vi "Find all vis in memory without documentation.vi"() -> ()   [LabVIEW 2010]
doc: "This .vi searches all .vi's in memory and returns the ones that do not have documentation. The .vis that are controls, in the .vi lib are ignored. The control on the front panel allows these .vis to be openned."
panel:
  in  "State":T1(ring)=enum."Minimized"
  out "Vis checked":i32(slide) scale=0.0..974.0
  in  "Open FPs of VI's without Documentation?":bool
  out "Total # without doc":i32
  out "Files without Documentation":string[](array[string])
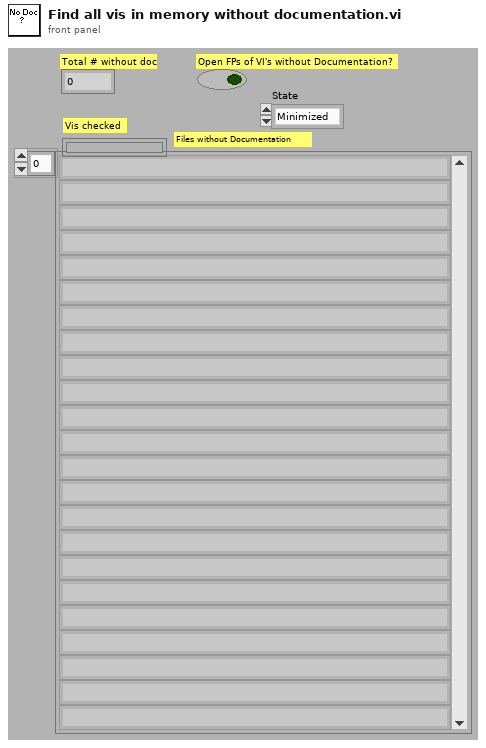
[diagram p1: front panel]
types:
  T1 = enum32{"Invalid", "Standard", "Closed", "Hidden", "Minimized", "Maximized"}
  T2 = enum32{"invalid VI type", "Standard VI", "Control VI", "Global VI", "Polymorphic VI", "Configuration VI", "SubSystem", "Facade VI", "Method VI", "Statechart Diagram VI"}
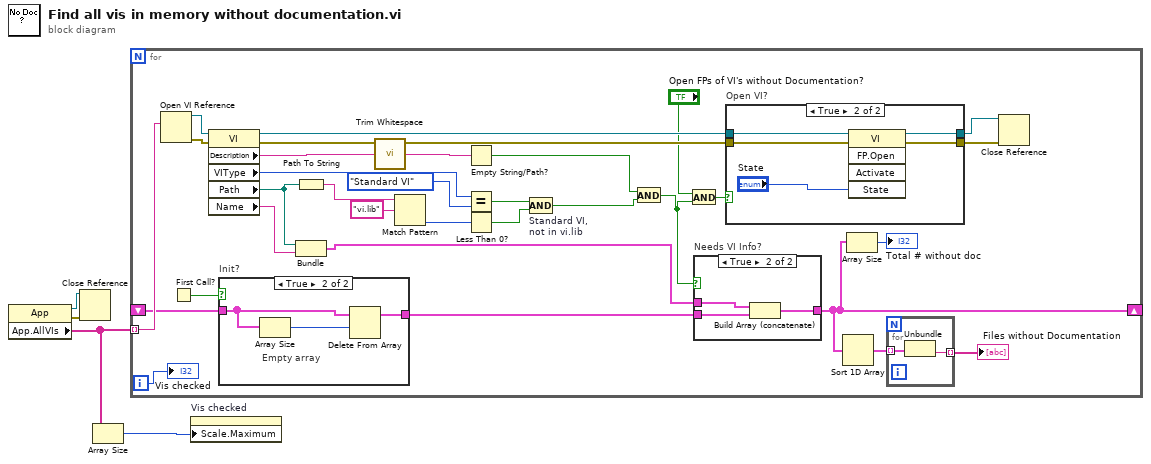
[diagram p0: block diagram]
diagram:
  n1 = property class="App"() -> (reference out=w1:refnum<vi>, error out=w2:errorcluster, "App.AllVIs"=w4:string[])  [unwired: 2 in]
  n2 = Close Reference(reference=w1, error in (no error)=w2) -> ()  [unwired: 1 out]
  n3 = Array Size(array=w4) -> (size(s)=w3:i32)
  n4 = for {
    tunnel: w4 -> [w31] mode=indexing
    shift-right: [w7] -> _
    shift-left: _ -> [w25]
    i -> [w15]
    n5 = Open VI Reference(vi path=w31) -> (vi reference=w36:refnum<vi>, error out=w35:errorcluster)  [unwired: 1 in, 4 out]
    n6 = First Call?() -> (First Call?: T/F=w23:bool)
    n7 = property class="VI"(reference=w36, error in=w35) -> (reference out=w22:refnum<vi>, error out=w21:errorcluster, "Description"=w13:string, "VIType"=w33:T2, "Path"=w14:path, "Name"=w9:string)
    n8 = case "Init?" shown="True" w23 {
      tunnel: w25 -> [w46 w49]
      tunnel: [w46 w47] -> w24
      frame False {
      }
      frame True {
        # "Empty array"
        n9 = Array Size(array=w49) -> (size(s)=w48:i32)
        n10 = Delete From Array(array=w49, length=w48) -> (array with subset deleted=w47:cluster{"Path":path, "Name":string}[])  [unwired: 1 in, 1 out]
      }
    }
    n11 = Path To String(path=w14) -> (string=w27:string)
    n12 = Bundle("Path"=w14, "Name"=w9) -> (w26:cluster{"Path":path, "Name":string})  [unwired: 1 out]
    n13 = call <vilib>:"Trim Whitespace.vi"("string"=w13) -> ("trimmed string"=w34:string)  [unwired: 1 in]
    n14 = Match Pattern(string=w27, regular expression="vi.lib") -> (offset past match=w29:i32)  [unwired: 4 out]
    n15 = Empty String/Path?(string/path=w34) -> (empty?=w12:bool)
    n16 = Equal?(x=w33, y=T2."Standard VI" ("VI Type")) -> (x = y?=w17:bool)
    n17 = Less Than 0?(x=w29) -> (x < 0?=w28:bool)
    n18 = Compound Arithmetic op=AND "Standard VI,\nnot in vi.lib"(w17, w28) -> (w10:bool)
    n19 = And(x=w12, y=w10) -> (x .and. y?=w11:bool)
    n20 = And(x="Open FPs of VI's without Documentation?", y=w11) -> (x .and. y?=w18:bool)
    n21 = case "Needs VI Info?" shown="True" w11 {
      tunnel: w24 -> [w50 w53]
      tunnel: [w50 w52] -> w7
      tunnel: w26 -> [_ w51]
      frame False {
      }
      frame True {
        n22 = Build Array (concatenate)(w51, w53) -> (w52:cluster{"Path":path, "Name":string}[])
      }
    }
    n23 = case "Open VI?" shown="True" w18 {
      tunnel: w22 -> [w39 w45]
      tunnel: w21 -> [w40 w44]
      tunnel: [w39 w43] -> w20
      tunnel: [w40 w42] -> w19
      frame False {
      }
      frame True {
        n24 = invoke class="VI" method="FP.Open"(reference=w45, error in=w44, "State"="State") -> (reference out=w43:refnum<vi>, error out=w42:errorcluster)  [unwired: 2 in, 3 out]
      }
    }
    n25 = Sort 1D Array(array=w7) -> (sorted array=w6:cluster{"Path":path, "Name":string}[])
    n26 = Array Size(array=w7) -> (size(s)=→"Total # without doc":i32)
    n27 = for {
      tunnel: w6 -> [w38] mode=indexing
      tunnel: [w37] -> w5 mode=indexing
      n28 = Unbundle(w38) -> ("Name"=w37:string)  [unwired: 1 out]
    }
    "Files without Documentation" <- w5
    n29 = Close Reference(reference=w20, error in (no error)=w19) -> ()  [unwired: 1 out]
    "Vis checked" <- w15
  }
  n30 = property on="Vis checked" class="Slide (strict)"("Scale.Maximum"=w3) -> ()  [unwired: 2 in, 2 out]
